vi "make_figure.vi"(6 "XX Array":dbl[](array[numeric]), 7 "X":i32, 9 "phase (rad)":dbl, 10 "b":i32, 11 "a":i32) -> (3 "data for display":cluster{dbl[], dbl[]})   [LabVIEW 2020]
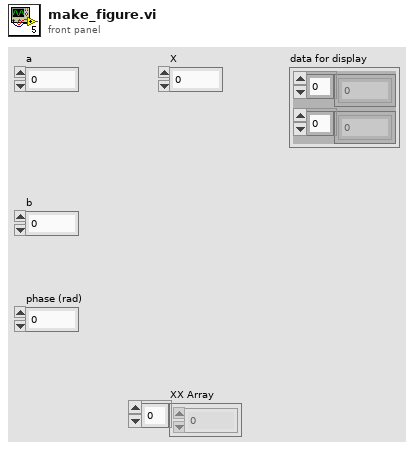
[diagram p1: front panel]
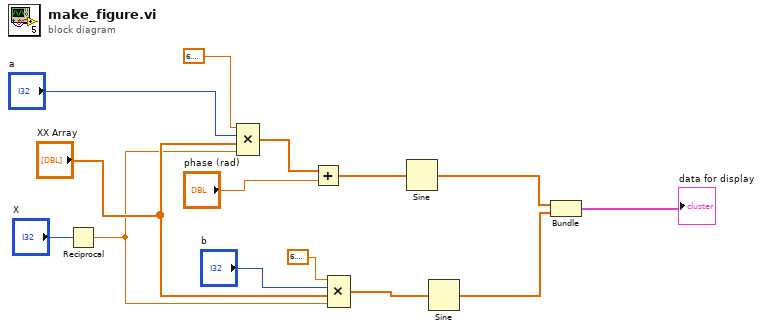
[diagram p0: block diagram]
diagram:
  n1 = Reciprocal(x="X") -> (1/x=w1:dbl)
  n2 = Compound Arithmetic op=MULTIPLY(6.283185307179586, "a", "XX Array", w1) -> (w8:dbl[])
  n3 = Add(x=w8, y="phase (rad)") -> (x+y=w10:dbl[])
  n4 = Compound Arithmetic op=MULTIPLY(6.283185307179586, "b", "XX Array", w1) -> (w11:dbl[])
  n5 = Sine(x=w10) -> (sin(x)=w12:dbl[])
  n6 = Sine(x=w11) -> (sin(x)=w13:dbl[])
  n7 = Bundle(w12, w13) -> (→"data for display":cluster{dbl[], dbl[]})  [unwired: 1 in]
